vi "Actor Last Ack Decorator.vi"(9 "Nest Error":errorcluster, 10 "Nest Actor":refnum<class "Actor.lvclass">, 11 "Dev Actor in":refnum<class "Dev Actor.lvclass">) -> (0 "error out":errorcluster, 3 "Dev Actor out":refnum<class "Dev Actor.lvclass">)   [LabVIEW 2021, in "Dev Actor.lvlib" / "Dev Actor.lvclass"]
uses:
  Dev Actor.lvclass
  LVCAM/LVCAM/Actor/Actor.lvclass
  Dev Actor.lvclass/Dev Actor.ctl
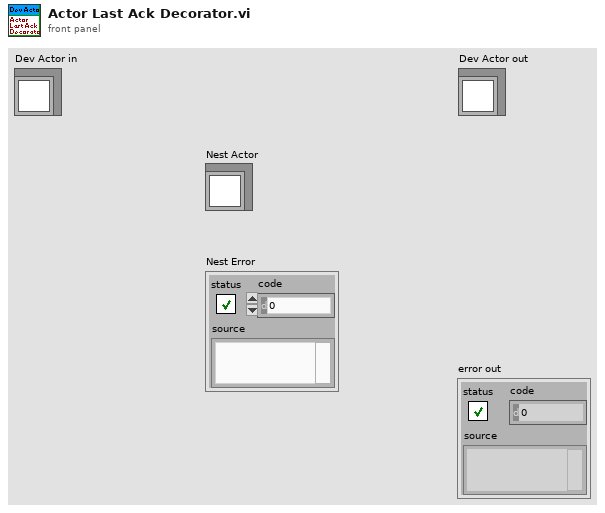
[diagram p1: front panel]
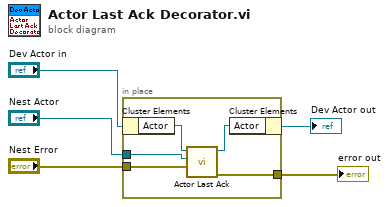
[diagram p0: block diagram]
diagram:
  n1 = in-place {
    in-place-border: "Nest Actor" -> [w8]
    in-place-border: [w7] -> w1
    in-place-border: "Nest Error" -> [w6]
    n2 = in-place-cluster #1("Dev Actor in") -> ("Actor"=w10:refnum<class "Actor.lvclass">)
    n3 = call-dynamic "Actor Last Ack.vi"("Nest Error"=w6, "Nest Actor"=w8, "Actor Last Ack in"=w10) -> ("error out"=w7:errorcluster, "Actor Last Ack out"=w9:refnum<class "Actor.lvclass">)  [unwired: 7 in]
    n4 = in-place-cluster #1("Actor"=w9) -> (→"Dev Actor out":refnum<class "Dev Actor.lvclass">)
  }
  "error out" <- w1
